vi "MainCleanUp.vi"   [LabVIEW 2020]
uses:
  <vilib>/Utility/config.llb/Read Key (String).vi
  <vilib>/Utility/config.llb/NI_LVConfig.lvlib
types:
  T1 = typedef "NI_LVConfig.lvlib/Config Data RefNum.ctl" = refnum<k1>
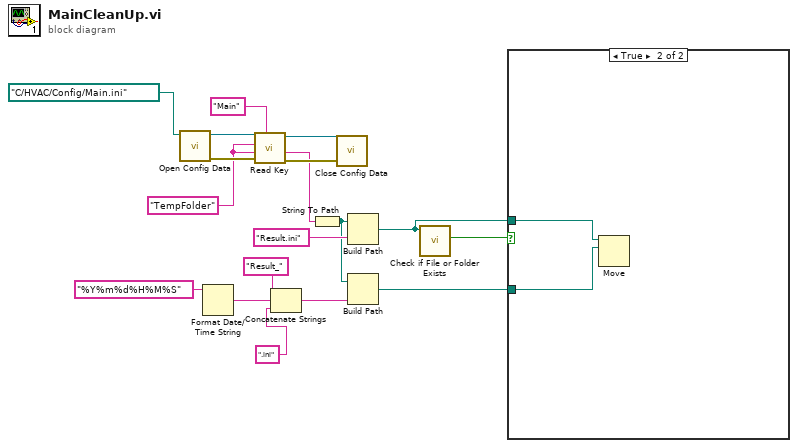
[diagram p0: block diagram]
diagram:
  w12 = "TempFolder" ("key")
  n1 = call <vilib>:"Open Config Data.vi"("configuration file path"=path "C:/HVAC/Config/Main.ini") -> ("error out"=w17:errorcluster, "refnum"=w16:T1)  [unwired: 8 in, 1 out]
  n2 = Format Date/Time String(time format string (%c)="%Y%m%d%H%M%S") -> (date/time string=w2:string)  [unwired: 2 in]
  n3 = call-poly <vilib>:"Read Key.vi"("section"="Main", "error in (no error)"=w17, "default value"=w12, "key"=w12, "refnum"=w16) -> ("error out"=w14:errorcluster, "value"=w11:string, "refnum out"=w15:T1)  [unwired: 3 in, 1 out]
  n4 = Concatenate Strings("Result_" ("string"), w2, ".ini" ("string")) -> (w6:string)
  n5 = String To Path(string=w11) -> (path=w7:path)
  n6 = call <vilib>:"Close Config Data.vi"("error in (no error)"=w14, "refnum"=w15) -> ()  [unwired: 8 in, 2 out]
  n7 = Build Path(base path=w7, name or relative path="Result.ini") -> (appended path=w8:path)
  n8 = Build Path(base path=w7, name or relative path=w6) -> (appended path=w1:path)
  n9 = call <vilib>:"Check if File or Folder Exists.vi"("path"=w8) -> ("file or folder exists?"=w9:bool)  [unwired: 8 in, 2 out]
  n10 = case shown="True" w9 {
    tunnel: w8 -> [_ w20]
    tunnel: w1 -> [_ w19]
    frame False {
    }
    frame True {
      n11 = Move(source path=w20, 10:w19) -> ()  [unwired: 3 in, 3 out]
    }
  }
